vi "Initialize UI.vi"(11 "Car Wash Display in":refnum<class "Car Wash Display.lvclass">) -> (3 "Car Wash Display out":refnum<class "Car Wash Display.lvclass">)   [LabVIEW 2016, in "CLD Exam - Car Wash.lvlib" / "Car Wash Display.lvclass"]
uses:
  Car Wash Display.lvclass
  Car Wash Display.lvclass/Car Wash Display.ctl
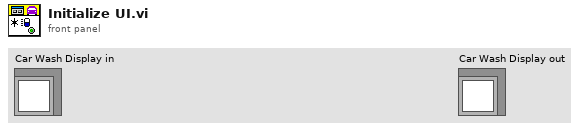
[diagram p1: front panel]
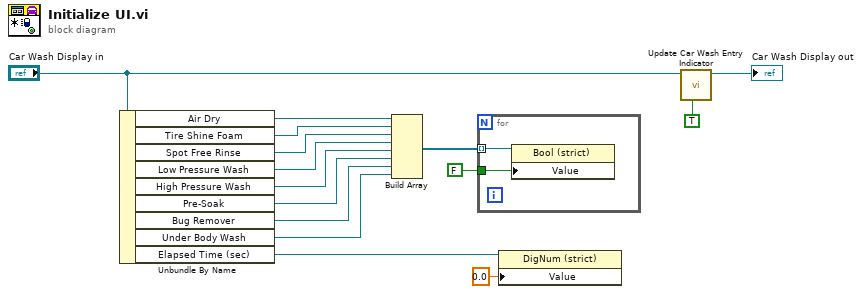
[diagram p0: block diagram]
diagram:
  n1 = Unbundle By Name("Car Wash Display in") -> ("Air Dry"=w15:refnum<vi>, "Tire Shine Foam"=w14:refnum<vi>, "Spot Free Rinse"=w13:refnum<vi>, "Low Pressure Wash"=w12:refnum<vi>, "High Pressure Wash"=w11:refnum<vi>, "Pre-Soak"=w10:refnum<vi>, "Bug Remover"=w9:refnum<vi>, "Under Body Wash"=w8:refnum<vi>, "Elapsed Time (sec)"=w5:refnum<vi>)
  n2 = Build Array(w15, w14, w13, w12, w11, w10, w9, w8) -> (w7:refnum<vi>[])
  n3 = for {
    tunnel: w7 -> [w17] mode=indexing
    tunnel: FALSE -> [w16]
    n4 = property class="Bool (strict)"(reference=w17, "Value"=w16) -> ()  [unwired: 1 in, 2 out]
  }
  n5 = property class="DigNum (strict)"(reference=w5, "Value"=0.0) -> ()  [unwired: 1 in, 2 out]
  n6 = call "Update Car Wash Entry Indicator.vi"("Vacant?"=TRUE, "Car Wash Display in"="Car Wash Display in") -> ("Car Wash Display out"=→"Car Wash Display out":refnum<class "Car Wash Display.lvclass">)  [unwired: 9 in]
